vi "Clear Entire Selection Lists.vi"   [LabVIEW 2023]
doc: "Demonstrates the use of the Clear Selection method in VI Scripting to clear the current selection on the front panel or block diagram."
panel:
  # "Overview: Demonstrates the use of the Clear Selection method in VI Scripting to clear the current selection on the front panel or block diagram.\nInstructions:\n1. Open Test - Selection List Target.vi.\n2. Select one or more objects on the front panel or block diagram.\n3. Run this VI. Whatever selection you previously made will be cleared. To see this, click the front panel or block diagram window title bar of the Test - Selection List Target.vi after running this VI to make it the active window."
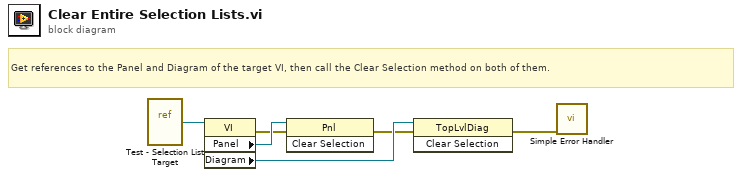
[diagram p0: block diagram]
diagram:
  # "Get references to the Panel and Diagram of the target VI, then call the Clear Selection method on both of them."
  n1 = vi-ref "Test - Selection List Target.vi"() -> (w6:refnum<vi>)
  n2 = property class="VI"(reference=w6) -> (error out=w3:errorcluster, "Panel"=w5:refnum<vi>, "Diagram"=w4:refnum<vi>)  [unwired: 1 in, 1 out]
  n3 = invoke class="Pnl" method="Clear Selection"(reference=w5, error in=w3) -> (error out=w2:errorcluster)  [unwired: 1 in, 2 out]
  n4 = invoke class="TopLvlDiag" method="Clear Selection"(reference=w4, error in=w2) -> (error out=w1:errorcluster)  [unwired: 1 in, 2 out]
  n5 = call <vilib>:"Simple Error Handler.vi"("error in (no error)"=w1) -> ()  [unwired: 4 in, 5 out]
